vi "drawpath.vi"(9 "new picture in":picture, 10 "reference in":refnum<vi>, 11 "Digital in":refnum<vi>) -> (3 "new picture":picture)   [LabVIEW 2016]
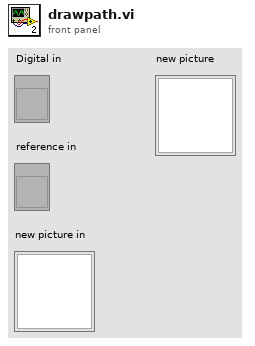
[diagram p1: front panel]
types:
  T1 = cluster{"Width":u16, "Style":enum32{"Solid", "Dash", "Dot", "DashDot", "DashDotDot"}}
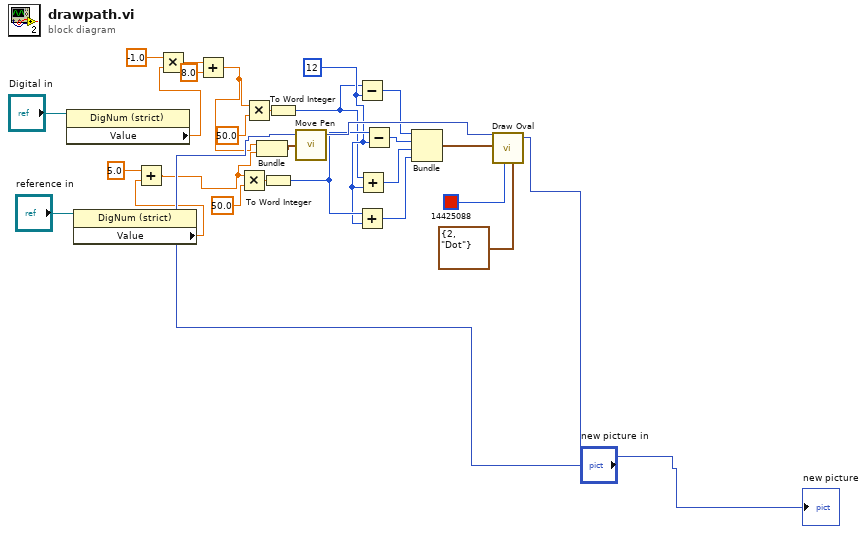
[diagram p0: block diagram]
diagram:
  w18 = i16 12 ("Waypoint \nSize")
  n1 = property class="DigNum (strict)"(reference="Digital in") -> ("Value"=w7:dbl)  [unwired: 1 in, 2 out]
  n2 = property class="DigNum (strict)"(reference="reference in") -> ("Value"=w2:dbl)  [unwired: 1 in, 2 out]
  n3 = Add(x=5.0, y=w2) -> (x+y=w3:dbl)
  n4 = Multiply(x=-1.0, y=w7) -> (x*y=w8:dbl)
  n5 = Add(x=w8, y=8.0) -> (x+y=w4:dbl)
  n6 = Multiply(x=w3, y=50.0) -> (x*y=w19:dbl)
  n7 = Multiply(x=w4, y=50.0) -> (x*y=w16:dbl)
  n8 = Bundle(w4, w3) -> (w24:cluster{dbl, dbl})  [unwired: 1 in]
  n9 = To Word Integer(number=w19) -> (16bit integer=w21:i16)
  n10 = To Word Integer(number=w16) -> (16bit integer=w17:i16)
  n11 = call <vilib>:"Move Pen.vi"("new position"=w24, "picture"="new picture in") -> ("new picture"=w25:picture)  [unwired: 3 in]
  n12 = Subtract(x=w17, y=w18) -> (x-y=w11:i16)
  n13 = Add(x=w21, y=w18) -> (x+y=w14:i16)
  n14 = Add(x=w17, y=w18) -> (x+y=w13:i16)
  n15 = Subtract(x=w21, y=w18) -> (x-y=w12:i16)
  n16 = Bundle(w11, w12, w13, w14) -> (w23:cluster{i16, i16, i16, i16})  [unwired: 1 in]
  n17 = call <vilib>:"Draw Oval.vi"("picture"=w25, "rect"=w23, "color(black)"=u32 14425088, "pen"=T1 {"Width"=2, "Style"=enum."Dot"}) -> ("new picture"=→"new picture":picture)  [unwired: 5 in]
